vi "Main Glue UI.vi"() -> ()   [LabVIEW 2011]
uses:
  C:/Program Files (x86)/National Instruments/LabVIEW 2011/user.lib/aerotech/8.2/Bin/Aerotech.A3200.dll
  Program Files (x86)/National Instruments/LabVIEW 2011/user.lib/aerotech/8.2/Bin/Aerotech.A3200.dll
  UI typedefs/Glue Progress Bar.ctl
  Potting Application/UI typedefs/Controller Commands.ctl
  UI typedefs/Glue Progress States.ctl
  Shared Components/WorkTable Class/Type Definitions/Worktable_Mode.ctl
  Shared Components/Gantry Class/Gantry Class.lvclass
  Application Utilities/Console Log/Console Log.lvclass
  Procedure Classes/Gluing Procedure/Gluing Procedure.lvclass
panel:
  out "error out":errorcluster
  out "Progress":T1 scale=0.0..7.0
  in  "Comment":string
  out "Console":string
  in  "Add Comment":bool
  in  "Resume Button":bool
  in  "Suspend Button":bool
  in  "Previous Button":bool
  in  "Execute Step":bool
  in  "Manual Control":bool
  in  "Emergency Stop":bool
  in  "ESTOP References":T2
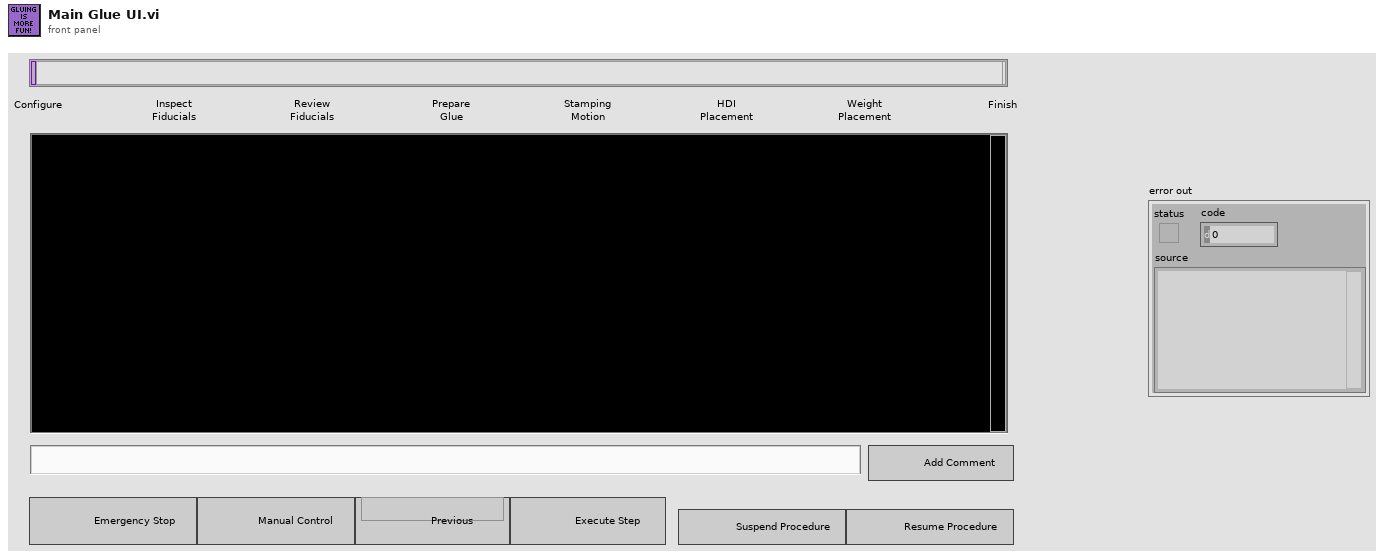
[diagram p1: front panel]
types:
  T1 = typedef "Glue Progress Bar.ctl" = u16
  T2 = cluster{"Aerotech Controller":refnum<k24>, "Manifold Task":refnum<k21>, "Dispenser Task":refnum<k21>}
  T3 = typedef "Glue Progress States.ctl" = enum16{"Configure", "Inspect Fuducials", "Review Fuducials", "Prepare Glue", "Stamping", "HDI Placement", "Weight Placement", "Finish"}
  T4 = typedef "Controller Commands.ctl" = enum16{"Initialize", "Execute Step", "Previous Step", "Add Comment", "Manual Control", "Resume", "Pause", "Emergency Stop"}
  T5 = cluster{"Aerotech Controller":refnum<k24>, "Dispenser IO Task":refnum<k21>, "Manifold IO Task":refnum<k21>}
  T6 = enum8{"Enabled", "Disabled", "Disabled and Grayed Out"}
  T7 = typedef "Worktable_Mode.ctl" = enum16{"Encapsulation", "Gluing"}
  T8 = enum16{"Left Button", "Center Button", "Right Button", "Window Close"}
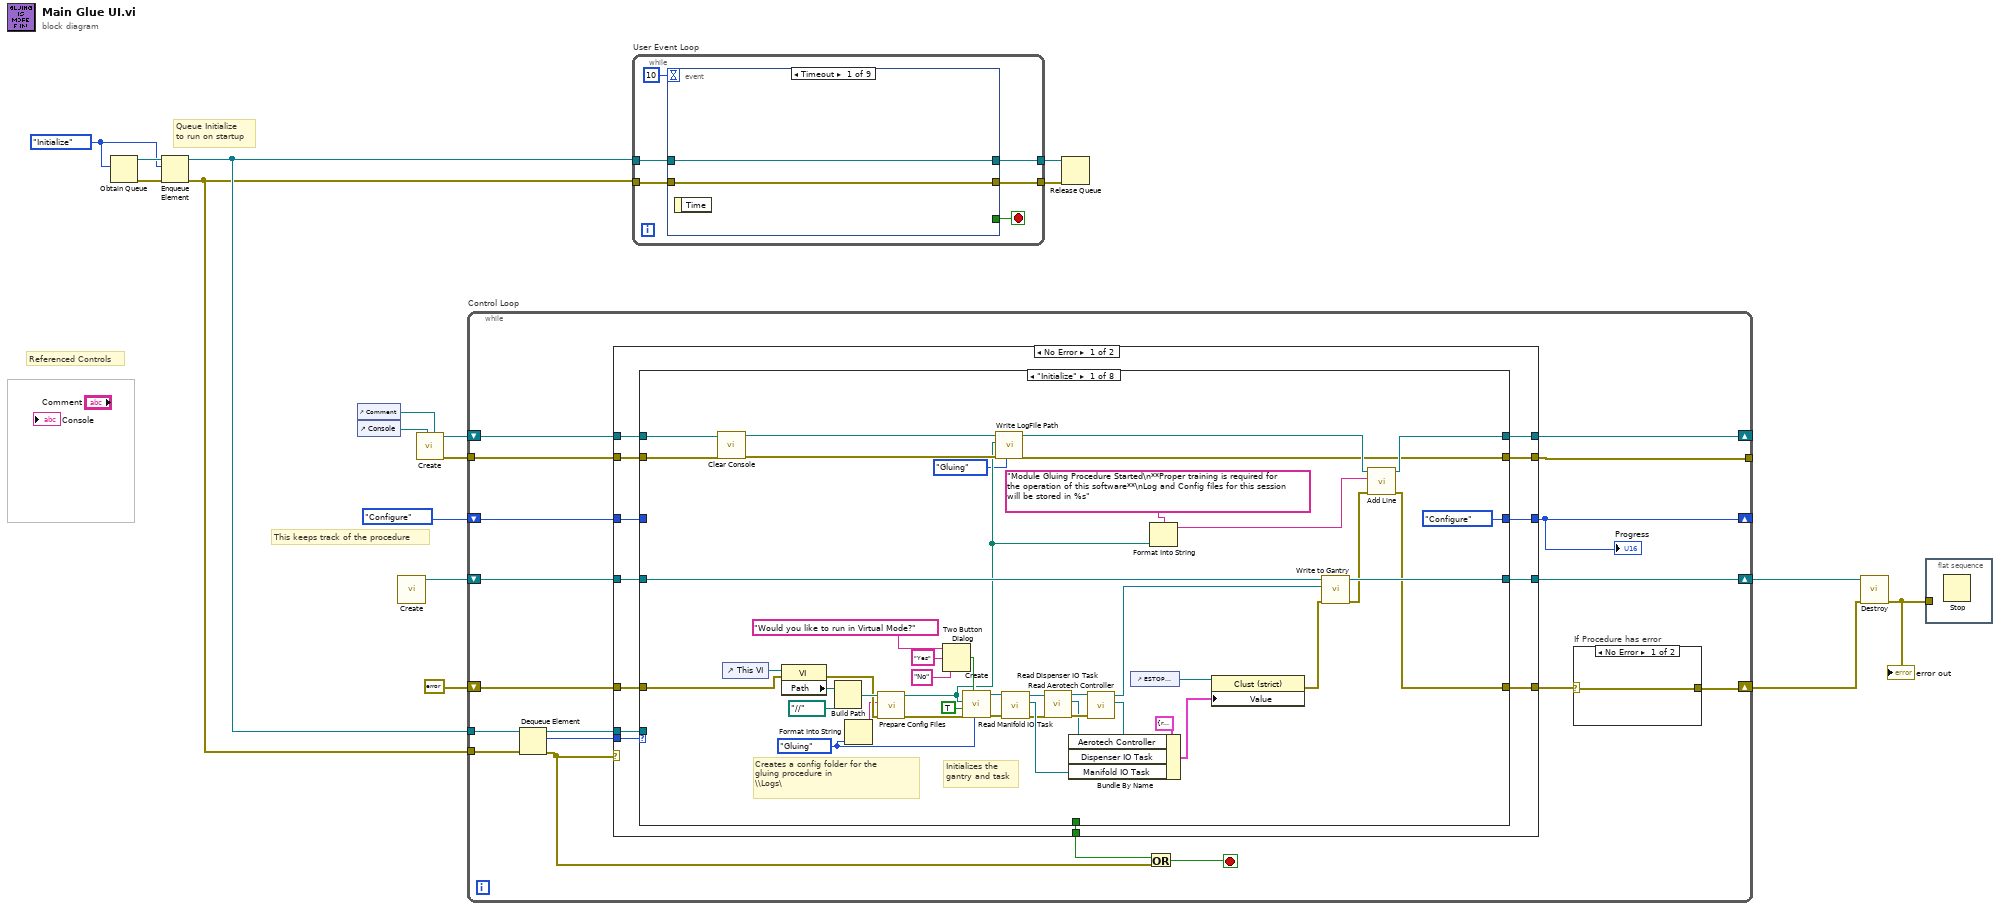
[diagram p0: block diagram]
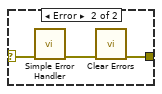
[diagram p2: hidden frame]
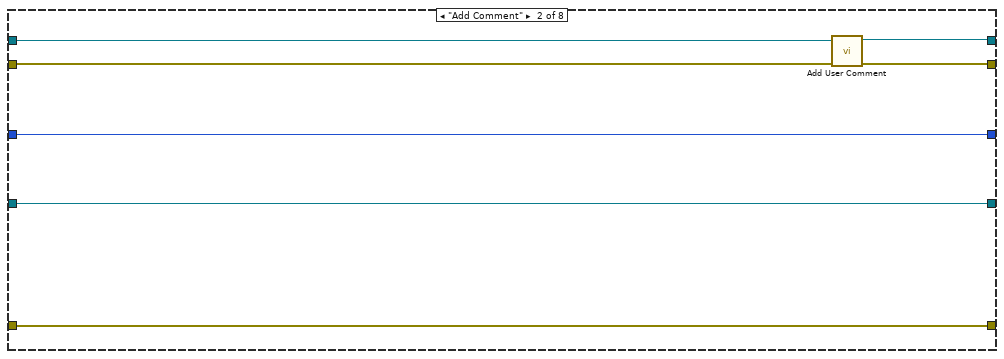
[diagram p3: hidden frame]
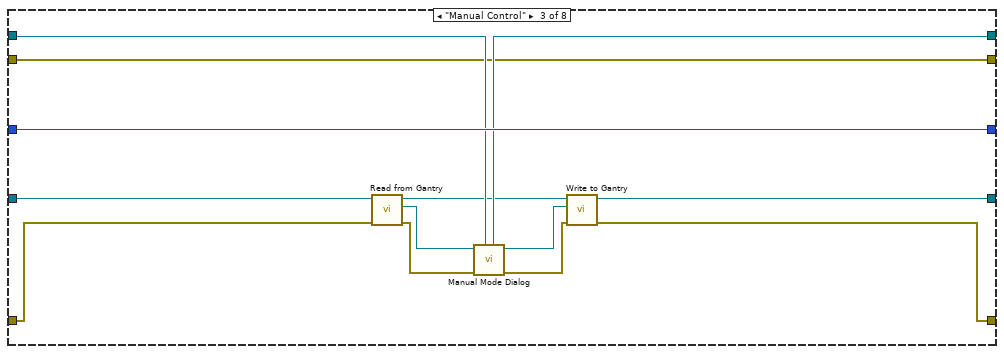
[diagram p4: hidden frame]
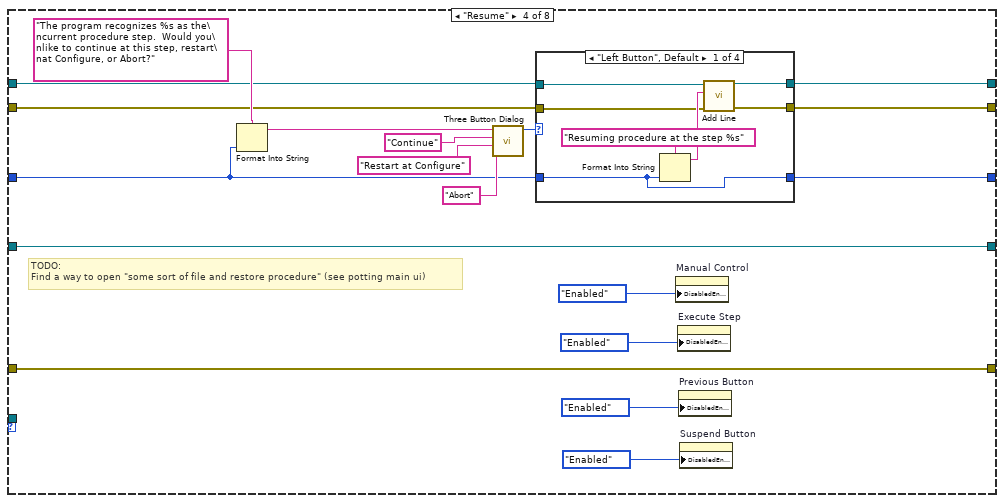
[diagram p5: hidden frame]
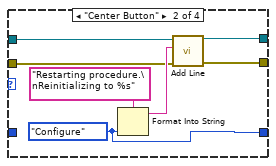
[diagram p6: hidden frame]
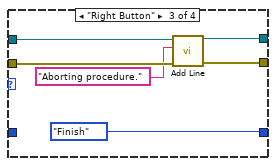
[diagram p7: hidden frame]
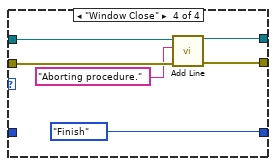
[diagram p8: hidden frame]
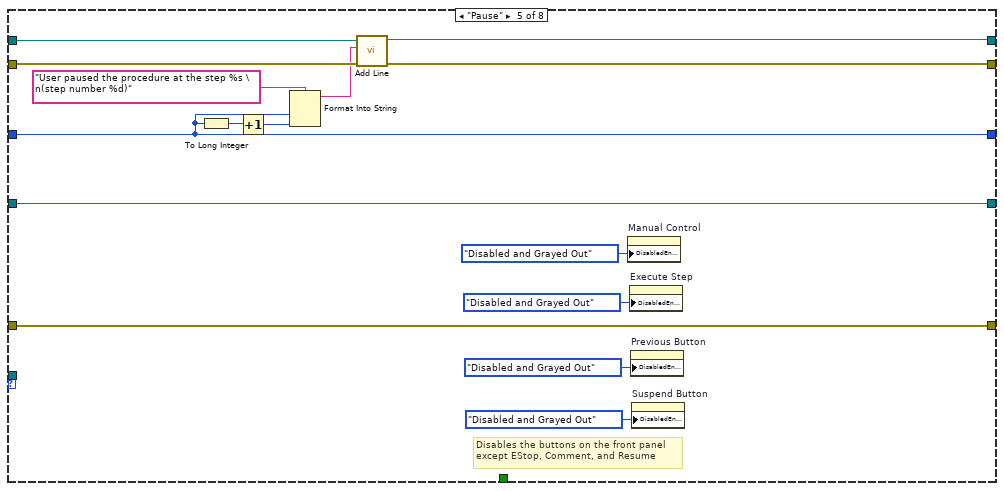
[diagram p9: hidden frame]
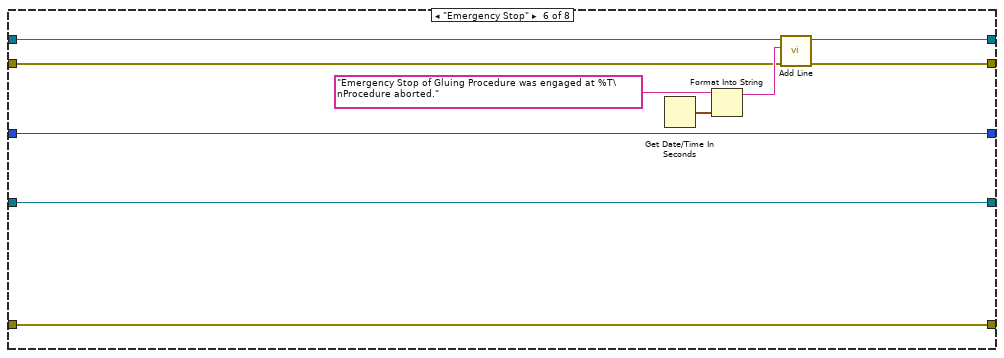
[diagram p10: hidden frame]
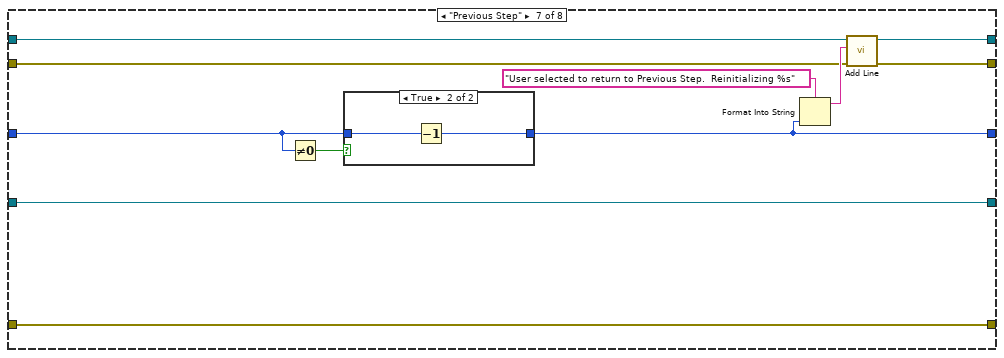
[diagram p11: hidden frame]
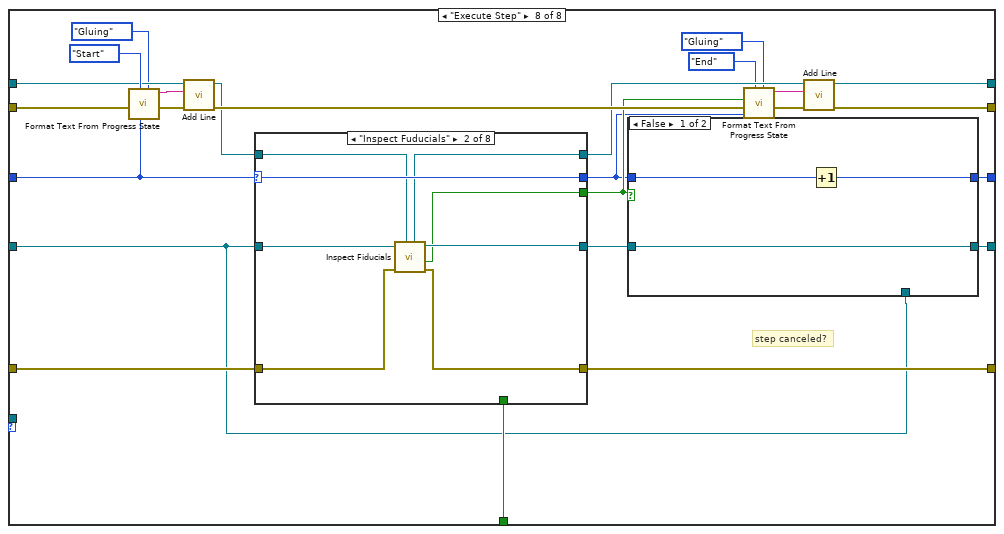
[diagram p13: hidden frame]
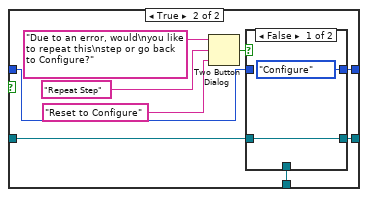
[diagram p14: hidden frame]
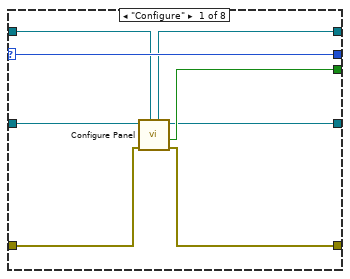
[diagram p16: hidden frame]
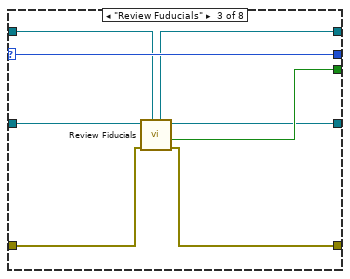
[diagram p17: hidden frame]
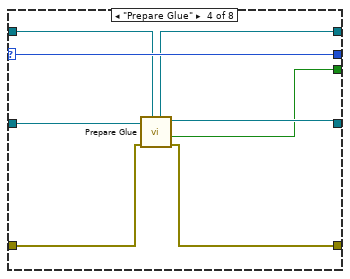
[diagram p18: hidden frame]
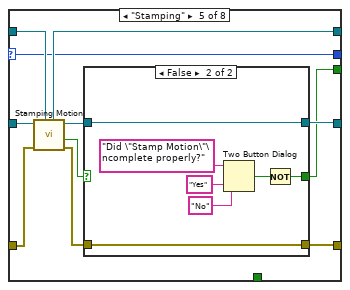
[diagram p19: hidden frame]
diagram:
  w13 = Controller_Commands."Initialize" ("Commands")
  # "This keeps track of the procedure"
  # "Referenced Controls"
  # "Queue Initialize \nto run on startup"
  n1 = Obtain Queue(element data type=w13) -> (queue out=w15:refnum<queue>, error out=w14:errorcluster)  [unwired: 4 in, 1 out]
  n2 = Enqueue Element(queue=w15, element=w13, error in (no error)=w14) -> (queue out=w7:refnum<queue>, error out=w6:errorcluster)  [unwired: 1 in, 1 out]
  n3 = control-ref of="Comment"() -> (w12:refnum<vi>)
  n4 = control-ref of="Console"() -> (w11:refnum<vi>)
  n5 = call "Create.vi"() -> ("Gluing Procedure out"=w1:refnum<class "Gluing Procedure.lvclass">)  [unwired: 10 in, 1 out]
  n6 = call "Create.vi"("Comment"=w12, "Console"=w11) -> ("error out"=w9:errorcluster, "Console Log out"=w10:refnum<class "Console Log.lvclass">)  [unwired: 8 in]
  n7 = while "Control Loop" {
    tunnel: w9 -> [w28]
    shift-right: [w20] -> _
    shift-left: w10 -> [w29]
    shift-right: [w19] -> _
    shift-left: Glue_Progress_States."Configure" ("Enum") -> [w27]
    shift-right: [w22] -> w4
    shift-left: w1 -> [w30]
    shift-right: [w23] -> w2
    shift-left: errorcluster {"status"=FALSE, "code"=0, "source"=""} ("error constant") -> [w31]
    tunnel: w7 -> [w34]
    tunnel: w6 -> [w35]
    tunnel: [w21] -> _
    stop <- w25 stop-if-true
    n8 = Dequeue Element(queue=w34, error in (no error)=w35) -> (queue out=w32:refnum<queue>, element=w33:T4, error out=w26:errorcluster)  [unwired: 1 in, 1 out]
    n9 = case shown="No Error" w26 {
      tunnel: w33 -> [w51 _]
      tunnel: w32 -> [w41 _]
      tunnel: w31 -> [w45 w341]
      tunnel: w30 -> [w46 w342]
      tunnel: w29 -> [w50 w345]
      tunnel: w28 -> [w48 w344]
      tunnel: w27 -> [w52 w343]
      tunnel: [w49 w345] -> w20
      tunnel: [w47 w344] -> w21
      tunnel: [w44 w341] -> w24
      tunnel: [w43 w342] -> w22
      tunnel: [w42 w343] -> w19
      tunnel: [w40 _] -> w18
      frame No Error {
        n10 = case shown="\"Initialize\"" w51 {
          tunnel: w52 -> [_ w103 w116 w124 w167 w185 w195 w212]
          tunnel: w50 -> [w67 w100 w114 w122 w173 w180 w188 w210]
          tunnel: [w63 w99 w115 w131 w169 w182 w192 w207] -> w49
          tunnel: w48 -> [w66 w97 w104 w123 w172 w176 w189 w219]
          tunnel: [w53 w98 w104 w117 w168 w181 w191 w219] -> w47
          tunnel: [Glue_Progress_States."Configure" ("Enum") w103 w116 w132 w167 w185 w187 w218] -> w42
          tunnel: [w69 w102 w105 w134 w175 w184 w194 w214] -> w43
          tunnel: w46 -> [w72 w102 w113 w134 w175 w184 w194 w213]
          tunnel: [w54 w101 w106 w133 w174 w183 w193 w217] -> w44
          tunnel: w45 -> [w95 w101 w107 w133 w174 w183 w193 w220]
          tunnel: w41 -> [_ _ _ _ _ _ _ _]
          tunnel: [_ _ _ _ _ _ _ w216] -> w40
          frame "Initialize" {
            w57 = Worktable_Mode."Gluing" ("Worktable Mode")
            # "Initializes the\ngantry and task"
            # "Creates a config folder for the\ngluing procedure in \n\\\\Logs\\"
            n11 = call "Clear Console.vi"("error in (no error)"=w66, "Console Log in"=w67) -> ("error out"=w64:errorcluster, "Console Log out"=w65:refnum<class "Console Log.lvclass">)  [unwired: 8 in]
            n12 = control-ref of="This VI"() -> (w96:refnum<vi>)
            n13 = property class="VI"(reference=w96, error in=w95) -> (error out=w91:errorcluster, "Path"=w94:path)  [unwired: 1 out]
            n14 = Build Path(base path=w94, name or relative path=path "../../..") -> (appended path=w92:path)
            n15 = Format Into String(w57) -> (resulting string=w56:string)  [unwired: 3 in, 1 out]
            n16 = call "Prepare Config Files.vi"("error in"=w91, "Config Prefix"=w56, "Project Root"=w92) -> ("error out"=w89:errorcluster, "Config Directory"=w59:path)  [unwired: 7 in]
            n17 = Two Button Dialog(message="Would you like to run in Virtual Mode?", 1:"No" ("F button name (\"Cancel\")"), 2:"Yes" ("T button name (\"OK\")")) -> (T button?=w88:bool)
            n18 = call "Create.vi"("Worktable Mode"=w57, "Virtual Mode"=w88, "error in"=w89, "HOME?"=TRUE, "Config Folder"=w59) -> ("error out"=w83:errorcluster, "Gantry out"=w84:refnum<class "Gantry Class.lvclass">)  [unwired: 5 in]
            n19 = call-dynamic "Write LogFile Path.vi"("Procedure Type"=enum16{"Potting", "Gluing"}."Gluing", "error in"=w64, "LogFile Directory"=w59, "Console Log in"=w65) -> ("error out"=w53:errorcluster, "Console Log out"=w62:refnum<class "Console Log.lvclass">)  [unwired: 6 in]
            n20 = call-dynamic "Read Manifold IO Task.vi"("error in (no error)"=w83, "Gantry Class in"=w84) -> ("error out"=w80:errorcluster, "Manifold IO Task"=w81:refnum<k21>, "Gantry Class out"=w82:refnum<class "Gantry Class.lvclass">)  [unwired: 7 in]
            n21 = call-dynamic "Read Dispenser IO Task.vi"("error in (no error)"=w80, "Gantry Class in"=w82) -> ("error out"=w78:errorcluster, "Dispenser IO Task"=w75:refnum<k21>, "Gantry Class out"=w79:refnum<class "Gantry Class.lvclass">)  [unwired: 7 in]
            n22 = call-dynamic "Read Aerotech Controller.vi"("error in (no error)"=w78, "Gantry Class in"=w79) -> ("Aerotech Controller"=w77:refnum<k24>, "Gantry Class out"=w71:refnum<class "Gantry Class.lvclass">)  [unwired: 7 in, 1 out]
            n23 = Bundle By Name(cluster=T5 {"Aerotech Controller"=refnum, "Dispenser IO Task"="", "Manifold IO Task"=""} ("input cluster"), "Aerotech Controller"=w77, "Dispenser IO Task"=w75, "Manifold IO Task"=w81) -> (w73:T5)
            n24 = control-ref of="ESTOP References"() -> (w74:refnum<vi>)
            n25 = Format Into String(format string="Module Gluing Procedure Started\n**Proper training is required for the operation of this software**\nLog and Config files for this session will be stored in %s" ("String"), w59) -> (resulting string=w61:string)  [unwired: 2 in, 1 out]
            n26 = property class="Clust (strict)"(reference=w74, "Value"=w73) -> (error out=w70:errorcluster)  [unwired: 1 in, 1 out]
            n27 = call "Write to Gantry.vi"("error in (no error)"=w70, "Gantry"=w71, "Gluing Procedure in"=w72) -> ("error out"=w55:errorcluster, "Gluing Procedure out"=w69:refnum<class "Gluing Procedure.lvclass">)  [unwired: 7 in]
            n28 = call "Add Line.vi"("error in"=w55, "String"=w61, "Console Log in"=w62) -> ("error out"=w54:errorcluster, "Console Log out"=w63:refnum<class "Console Log.lvclass">)  [unwired: 7 in]
          }
          frame "Add Comment" {
            n29 = call "Add User Comment.vi"("error in"=w97, "Console Log in"=w100) -> ("error out"=w98:errorcluster, "Console Log out"=w99:refnum<class "Console Log.lvclass">)  [unwired: 8 in]
          }
          frame "Manual Control" {
            n30 = call "Read from Gantry.vi"("error in (no error)"=w107, "Gluing Procedure in"=w113) -> ("error out"=w110:errorcluster, "Gantry"=w112:refnum<class "Gantry Class.lvclass">, "Gluing Procedure out"=w108:refnum<class "Gluing Procedure.lvclass">)  [unwired: 7 in]
            n31 = call "Manual Mode Dialog.vi"("Console Log in"=w114, "error in"=w110, "Gantry in"=w112) -> ("error out"=w109:errorcluster, "Gantry out"=w111:refnum<class "Gantry Class.lvclass">, "Console Log out"=w115:refnum<class "Console Log.lvclass">)  [unwired: 6 in]
            n32 = call "Write to Gantry.vi"("error in (no error)"=w109, "Gantry"=w111, "Gluing Procedure in"=w108) -> ("error out"=w106:errorcluster, "Gluing Procedure out"=w105:refnum<class "Gluing Procedure.lvclass">)  [unwired: 7 in]
          }
          frame "Resume" {
            # "TODO:\nFind a way to open \"some sort of file and restore procedure\" (see potting main ui)"
            n33 = Format Into String(format string="The program recognizes %s as the\ncurrent procedure step.  Would you\nlike to continue at this step, restart\nat Configure, or Abort?" ("Window Title (\"\")"), w124) -> (resulting string=w128:string)  [unwired: 2 in, 1 out]
            n34 = call <vilib>:"Three Button Dialog.vi"("Right Button Text (\"Cancel\")"="Abort" ("Right Button Text (\"Cancel\")"), "Center Button Text (\"No\")"="Restart at Configure" ("Center Button Text (\"No\")"), "Left Button Text (\"Yes\")"="Continue" ("Left Button Text (\"Yes\")"), "message"=w128) -> ("Which Button?"=w130:T8)  [unwired: 7 in]
            n35 = case shown="\"Left Button\", Default" w130 {
              tunnel: [w141 w145 w153 w159] -> w131
              tunnel: [w140 w146 w154 w160] -> w117
              tunnel: w124 -> [w135 _ _ _]
              tunnel: w123 -> [w137 w143 w151 w157]
              tunnel: w122 -> [w136 w144 w152 w158]
              tunnel: [w135 w142 Glue_Progress_States."Finish" ("Enum") Glue_Progress_States."Finish" ("Enum")] -> w132
              frame "Left Button", Default {
                n36 = Format Into String(format string="Resuming procedure at the step %s", w135) -> (resulting string=w139:string)  [unwired: 2 in, 1 out]
                n37 = call "Add Line.vi"("error in"=w137, "String"=w139, "Console Log in"=w136) -> ("error out"=w140:errorcluster, "Console Log out"=w141:refnum<class "Console Log.lvclass">)  [unwired: 7 in]
              }
              frame "Center Button" {
                w142 = Glue_Progress_States."Configure" ("Enum")
                n38 = Format Into String(format string="Restarting procedure.\nReinitializing to %s", w142) -> (resulting string=w147:string)  [unwired: 2 in, 1 out]
                n39 = call "Add Line.vi"("error in"=w143, "String"=w147, "Console Log in"=w144) -> ("error out"=w146:errorcluster, "Console Log out"=w145:refnum<class "Console Log.lvclass">)  [unwired: 7 in]
              }
              frame "Right Button" {
                n40 = call "Add Line.vi"("error in"=w151, "String"="Aborting procedure." ("format string"), "Console Log in"=w152) -> ("error out"=w154:errorcluster, "Console Log out"=w153:refnum<class "Console Log.lvclass">)  [unwired: 7 in]
              }
              frame "Window Close" {
                n41 = call "Add Line.vi"("error in"=w157, "String"="Aborting procedure." ("format string"), "Console Log in"=w158) -> ("error out"=w160:errorcluster, "Console Log out"=w159:refnum<class "Console Log.lvclass">)  [unwired: 7 in]
              }
            }
            n42 = property on="Manual Control" class="Bool (strict)"("DisabledEnum"=T6."Enabled" ("Disabled")) -> ()  [unwired: 2 in, 2 out]
            n43 = property on="Execute Step" class="Bool (strict)"("DisabledEnum"=T6."Enabled" ("Disabled")) -> ()  [unwired: 2 in, 2 out]
            n44 = property on="Previous Button" class="Bool (strict)"("DisabledEnum"=T6."Enabled" ("Disabled")) -> ()  [unwired: 2 in, 2 out]
            n45 = property on="Suspend Button" class="Bool (strict)"("DisabledEnum"=T6."Enabled" ("Disabled")) -> ()  [unwired: 2 in, 2 out]
          }
          frame "Pause" {
            # "Disables the buttons on the front panel\nexcept EStop, Comment, and Resume"
            n46 = To Long Integer(number=w167) -> (32bit integer=w166:i32)
            n47 = Increment(x=w166) -> (x+1=w165:i32)
            n48 = Format Into String(format string="User paused the procedure at the step %s \n(step number %d)", w167, w165) -> (resulting string=w171:string)  [unwired: 2 in, 1 out]
            n49 = call "Add Line.vi"("error in"=w172, "String"=w171, "Console Log in"=w173) -> ("error out"=w168:errorcluster, "Console Log out"=w169:refnum<class "Console Log.lvclass">)  [unwired: 7 in]
            n50 = property on="Manual Control" class="Bool (strict)"("DisabledEnum"=T6."Disabled and Grayed Out" ("Disabled")) -> ()  [unwired: 2 in, 2 out]
            n51 = property on="Execute Step" class="Bool (strict)"("DisabledEnum"=T6."Disabled and Grayed Out" ("Disabled")) -> ()  [unwired: 2 in, 2 out]
            n52 = property on="Previous Button" class="Bool (strict)"("DisabledEnum"=T6."Disabled and Grayed Out" ("Disabled")) -> ()  [unwired: 2 in, 2 out]
            n53 = property on="Suspend Button" class="Bool (strict)"("DisabledEnum"=T6."Disabled and Grayed Out" ("Disabled")) -> ()  [unwired: 2 in, 2 out]
          }
          frame "Emergency Stop" {
            n54 = Get Date/Time In Seconds() -> (seconds since 1Jan1904=w178:timestamp)
            n55 = Format Into String(format string="Emergency Stop of Gluing Procedure was engaged at %T\nProcedure aborted.", w178) -> (resulting string=w179:string)  [unwired: 2 in, 1 out]
            n56 = call "Add Line.vi"("error in"=w176, "String"=w179, "Console Log in"=w180) -> ("error out"=w181:errorcluster, "Console Log out"=w182:refnum<class "Console Log.lvclass">)  [unwired: 7 in]
          }
          frame "Previous Step" {
            n57 = Not Equal To 0?(x=w195) -> (x != 0?=w196:bool)
            n58 = case shown="True" w196 {
              tunnel: w195 -> [w197 w199]
              tunnel: [w197 w198] -> w187
              frame False {
              }
              frame True {
                n59 = Decrement(x=w199) -> (x-1=w198:T3)
              }
            }
            n60 = Format Into String(format string="User selected to return to Previous Step.  Reinitializing %s", w187) -> (resulting string=w190:string)  [unwired: 2 in, 1 out]
            n61 = call "Add Line.vi"("error in"=w189, "String"=w190, "Console Log in"=w188) -> ("error out"=w191:errorcluster, "Console Log out"=w192:refnum<class "Console Log.lvclass">)  [unwired: 7 in]
          }
          frame "Execute Step" {
            # "step canceled?"
            n62 = call "Format Text From Progress State.vi"("Procedure type"=Worktable_Mode."Gluing", "Glue Procedure Steps"=w212, "Start/End"=enum16{"Start", "End"}."Start") -> ("String"=w209:string)  [unwired: 8 in]
            n63 = call "Add Line.vi"("String"=w209, "Console Log in"=w210) -> ("Console Log out"=w208:refnum<class "Console Log.lvclass">)  [unwired: 8 in, 1 out]
            n64 = case shown="\"Inspect Fuducials\"" w212 {
              selector: w212 -> [w244 w249 w259 w263 w276 w299 w320 w337]
              tunnel: w213 -> [w239 w252 w260 w268 w279 w300 w321 w340]
              tunnel: w220 -> [w238 w246 w254 w264 w275 w296 w317 w334]
              tunnel: w208 -> [w243 w248 w258 w262 w278 w298 w319 w339]
              tunnel: [_ _ _ _ _ _ _ TRUE] -> w216
              tunnel: [w244 w249 w259 w263 w276 w299 w320 w337] -> w202
              tunnel: [w242 w247 w257 w261 w277 w297 w318 w338] -> w205
              tunnel: [w240 w251 w255 w267 w273 w290 w315 w335] -> w215
              tunnel: [w237 w245 w253 w265 w272 w292 w311 w333] -> w217
              tunnel: [w241 w250 w256 w266 w269 w294 w314 w336] -> w203
              frame "Configure" {
                n65 = call "Configure Panel.vi"("Console Log in"=w243, "error in"=w238, "Gluing Procedure in"=w239) -> ("error out"=w237:errorcluster, "Cancel Button status"=w241:bool, "Gluing Procedure out"=w240:refnum<class "Gluing Procedure.lvclass">, "Console Log out"=w242:refnum<class "Console Log.lvclass">)  [unwired: 5 in]
              }
              frame "Inspect Fuducials" {
                n66 = call "Inspect Fiducials.vi"("Console Log in"=w248, "error in"=w246, "Gluing Procedure in"=w252) -> ("error out"=w245:errorcluster, "Step canceled?"=w250:bool, "Gluing Procedure out"=w251:refnum<class "Gluing Procedure.lvclass">, "Console Log out"=w247:refnum<class "Console Log.lvclass">)  [unwired: 5 in]
              }
              frame "Review Fuducials" {
                n67 = call "Review Fiducials.vi"("Console Log in"=w258, "error in"=w254, "Gluing Procedure in"=w260) -> ("error out"=w253:errorcluster, "Step canceled?"=w256:bool, "Gluing Procedure out"=w255:refnum<class "Gluing Procedure.lvclass">, "Console Log out"=w257:refnum<class "Console Log.lvclass">)  [unwired: 5 in]
              }
              frame "Prepare Glue" {
                n68 = call "Prepare Glue.vi"("Console Log in"=w262, "error in"=w264, "Gluing Procedure in"=w268) -> ("error out"=w265:errorcluster, "Step canceled?"=w266:bool, "Gluing Procedure out"=w267:refnum<class "Gluing Procedure.lvclass">, "Console Log out"=w261:refnum<class "Console Log.lvclass">)  [unwired: 5 in]
              }
              frame "Stamping" {
                n69 = call "Stamping Motion.vi"("Console Log in"=w278, "error in"=w275, "Gluing Procedure in"=w279) -> ("error out"=w271:errorcluster, "Step canceled?"=w270:bool, "Gluing Procedure out"=w274:refnum<class "Gluing Procedure.lvclass">, "Console Log out"=w277:refnum<class "Console Log.lvclass">)  [unwired: 5 in]
                n70 = case shown="False" w270 {
                  selector: w270 -> [w282 _]
                  tunnel: [w282 w286] -> w269
                  tunnel: w271 -> [w280 w284]
                  tunnel: [w280 w284] -> w272
                  tunnel: w274 -> [w281 w283]
                  tunnel: [w281 w283] -> w273
                  frame True {
                  }
                  frame False {
                    n71 = Two Button Dialog(message="Did \"Stamp Motion\"\ncomplete properly?", 1:"No" ("F button name (\"Cancel\")"), 2:"Yes" ("T button name (\"OK\")")) -> (T button?=w285:bool)
                    n72 = Not(x=w285) -> (.not. x?=w286:bool)
                  }
                }
              }
              frame "HDI Placement" {
                n73 = call "HDI Placement motion.vi"("Console Log in"=w298, "error in"=w296, "Gluing Procedure in"=w300) -> ("error out"=w293:errorcluster, "Step canceled?"=w295:bool, "Gluing Procedure out"=w291:refnum<class "Gluing Procedure.lvclass">, "Console Log out"=w297:refnum<class "Console Log.lvclass">)  [unwired: 5 in]
                n74 = case shown="False" w295 {
                  selector: w295 -> [w303 _]
                  tunnel: [w303 w307] -> w294
                  tunnel: w293 -> [w301 w305]
                  tunnel: [w301 w305] -> w292
                  tunnel: w291 -> [w302 w304]
                  tunnel: [w302 w304] -> w290
                  frame True {
                  }
                  frame False {
                    n75 = Two Button Dialog(message="Did \"HDI Placement\"\ncomplete properly?", 1:"No" ("F button name (\"Cancel\")"), 2:"Yes" ("T button name (\"OK\")")) -> (T button?=w306:bool)
                    n76 = Not(x=w306) -> (.not. x?=w307:bool)
                  }
                }
              }
              frame "Weight Placement" {
                n77 = call "Weight Motion.vi"("Console Log in"=w319, "error in"=w317, "Gluing Procedure in"=w321) -> ("error out"=w312:errorcluster, "Step canceled?"=w313:bool, "Gluing Procedure out"=w316:refnum<class "Gluing Procedure.lvclass">, "Console Log out"=w318:refnum<class "Console Log.lvclass">)  [unwired: 5 in]
                n78 = case shown="False" w313 {
                  selector: w313 -> [w324 _]
                  tunnel: [w324 w328] -> w314
                  tunnel: w312 -> [w322 w326]
                  tunnel: [w322 w326] -> w311
                  tunnel: w316 -> [w323 w325]
                  tunnel: [w323 w325] -> w315
                  frame True {
                  }
                  frame False {
                    n79 = Two Button Dialog(message="Did \"Weight Placement\"\ncomplete properly?", 1:"No" ("F button name (\"Cancel\")"), 2:"Yes" ("T button name (\"OK\")")) -> (T button?=w327:bool)
                    n80 = Not(x=w327) -> (.not. x?=w328:bool)
                  }
                }
              }
              frame "Finish" {
                n81 = call "Write Log Summary Dialog.vi"("Console Log in"=w339, "error in"=w334, "Gluing Procedure in"=w340) -> ("error out"=w333:errorcluster, "Step canceled?"=w336:bool, "Gluing Procedure out"=w335:refnum<class "Gluing Procedure.lvclass">, "Console Log out"=w338:refnum<class "Console Log.lvclass">)  [unwired: 5 in]
              }
            }
            n82 = case shown="False" w203 {
              tunnel: w202 -> [w223 w228]
              tunnel: [w222 w227] -> w218
              tunnel: w215 -> [w221 w226]
              tunnel: [w221 w225] -> w214
              tunnel: w213 -> [_ w224]
              frame False {
                n83 = Increment(x=w223) -> (x+1=w222:T3)
              }
              frame True {
                n84 = Two Button Dialog(message="Due to an error, would\nyou like to repeat this\nstep or go back to Configure?", 1:"Reset to Configure" ("F button name (\"Cancel\")"), 2:"Repeat Step" ("T button name (\"OK\")")) -> (T button?=w232:bool)
                n85 = case shown="False" w232 {
                  tunnel: w228 -> [_ w236]
                  tunnel: [Glue_Progress_States."Configure" ("Enum") w236] -> w227
                  tunnel: w226 -> [w233 _]
                  tunnel: [w233 w235] -> w225
                  tunnel: w224 -> [_ w235]
                  frame False {
                  }
                  frame True {
                  }
                }
              }
            }
            n86 = call "Format Text From Progress State.vi"("Procedure type"=Worktable_Mode."Gluing", "Glue Procedure Steps"=w202, "Start/End"=enum16{"Start", "End"}."End", "Canceled"=w203) -> ("String"=w206:string)  [unwired: 7 in]
            n87 = call "Add Line.vi"("String"=w206, "Console Log in"=w205) -> ("Console Log out"=w207:refnum<class "Console Log.lvclass">)  [unwired: 8 in, 1 out]
          }
        }
      }
      frame Error {
      }
    }
    "Progress" <- w19
    n88 = Or(x=w18, y=w26) -> (x .or. y?=w25:bool)
    n89 = case "If Procedure has error" shown="No Error" w24 {
      selector: w24 -> [w36 w39]
      tunnel: [w36 w38] -> w23
      frame No Error {
      }
      frame Error {
        n90 = call <vilib>:"Simple Error Handler.vi"("error in (no error)"=w39) -> ("error out"=w37:errorcluster)  [unwired: 4 in, 4 out]
        n91 = call <vilib>:"Clear Errors.vi"("error in (no error)"=w37) -> ("error out"=w38:errorcluster)  [unwired: 6 in]
      }
    }
  }
  n92 = while "User Event Loop" {
    tunnel: w7 -> [w346]
    tunnel: [w349] -> w17
    tunnel: w6 -> [w348]
    tunnel: [w347] -> w16
    stop <- w350 stop-if-true
    n93 = event shown="[0] Timeout" {
      selector: _ -> [_ _ _ _ _ _ _ _ _]
      dyn-events: _ -> [_ _ _ _ _ _ _ _ _]
      timeout: 10 -> [_ _ _ _ _ _ _ _ _]
      tunnel: [_ _ _ _ _ _ _ w384 _] -> w350
      tunnel: w346 -> [w353 w356 w360 w366 w368 w374 w379 w383 w390]
      tunnel: [w353 w356 w359 w363 w370 w376 w381 w383 w391] -> w349
      tunnel: w348 -> [w352 w355 w358 w365 w367 w373 w378 w382 w393]
      tunnel: [w352 w355 w357 w364 w369 w375 w377 w382 w392] -> w347
      event Timeout {
        n94 = event-data() -> ()  [unwired: 1 in, 1 out]
      }
      event "Emergency Stop": Mouse Up {
        n95 = event-data() -> ()  [unwired: 1 in, 1 out]
        n96 = call "Emergency Stop.vi"("ESTOP References"="ESTOP References") -> ()
      }
      event "Manual Control": Mouse Up {
        n97 = event-data() -> ()  [unwired: 1 in, 1 out]
        n98 = Enqueue Element(queue=w360, element=Controller_Commands."Manual Control", error in (no error)=w358) -> (queue out=w359:refnum<queue>, error out=w357:errorcluster)  [unwired: 1 in, 1 out]
      }
      event "Execute Step": Mouse Up {
        n99 = event-data() -> ()  [unwired: 1 in, 1 out]
        n100 = Enqueue Element(queue=w366, element=Controller_Commands."Execute Step", error in (no error)=w365) -> (queue out=w363:refnum<queue>, error out=w364:errorcluster)  [unwired: 1 in, 1 out]
      }
      event "Previous Button": Mouse Up {
        n101 = event-data() -> ()  [unwired: 1 in, 1 out]
        n102 = Enqueue Element(queue=w368, element=Controller_Commands."Previous Step", error in (no error)=w367) -> (queue out=w370:refnum<queue>, error out=w369:errorcluster)  [unwired: 1 in, 1 out]
      }
      event "Suspend Button": Mouse Up {
        n103 = event-data() -> ()  [unwired: 1 in, 1 out]
        n104 = Enqueue Element(queue=w374, element=Controller_Commands."Pause", error in (no error)=w373) -> (queue out=w376:refnum<queue>, error out=w375:errorcluster)  [unwired: 1 in, 1 out]
      }
      event "Resume Button": Mouse Up {
        n105 = event-data() -> ()  [unwired: 1 in, 1 out]
        n106 = Enqueue Element(queue=w379, element=Controller_Commands."Resume", error in (no error)=w378) -> (queue out=w381:refnum<queue>, error out=w377:errorcluster)  [unwired: 1 in, 1 out]
      }
      event Panel Close? {
        n107 = event-data() -> ()  [unwired: 1 in, 1 out]
        n108 = Two Button Dialog(message="Are you sure you want to quit?", 1:"Return" ("F button name (\"Cancel\")"), 2:"Quit" ("T button name (\"OK\")")) -> (T button?=w384:bool)
        n109 = event-data("Discard?"=TRUE) -> ()  [unwired: 1 in, 1 out]
      }
      event "Add Comment": Mouse Up {
        n110 = event-data() -> ()  [unwired: 1 in, 1 out]
        n111 = Enqueue Element(queue=w390, element=Controller_Commands."Add Comment", error in (no error)=w393) -> (queue out=w391:refnum<queue>, error out=w392:errorcluster)  [unwired: 1 in, 1 out]
      }
    }
  }
  n112 = Release Queue(queue=w17, error in (no error)=w16) -> ()  [unwired: 1 in, 3 out]
  n113 = call "Destroy.vi"("error in"=w2, "Gluing Procedure in"=w4) -> ("error out"=w3:errorcluster)  [unwired: 9 in]
  "error out" <- w3
  n114 = flat-sequence {
    tunnel: w3 -> [_]
    frame #0 {
      n115 = Stop() -> ()  [unwired: 1 in]
    }
  }
